vi "Configure Control.vi"(8 "error in (no error)":errorcluster, 10 "control":refnum<vi>, 11 "NT Enum in":refnum<class "NT Enum.lvclass">) -> (0 "error out":errorcluster, 2 "control out":refnum<vi>, 3 "NT Enum out":refnum<class "NT Enum.lvclass">)   [LabVIEW 2020, in "PV Access.lvlib" / "PV Data.lvlib" / "NT Enum.lvclass"]
doc: "Set the description of <B>control</B> from the value's metadata."
uses:
  NT Enum.lvclass
  NT Base/NT Base.lvclass
  NT Enum.lvclass/NT Enum.ctl
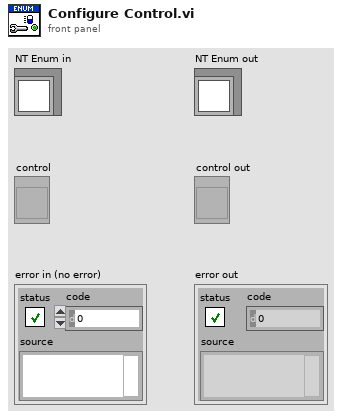
[diagram p1: front panel]
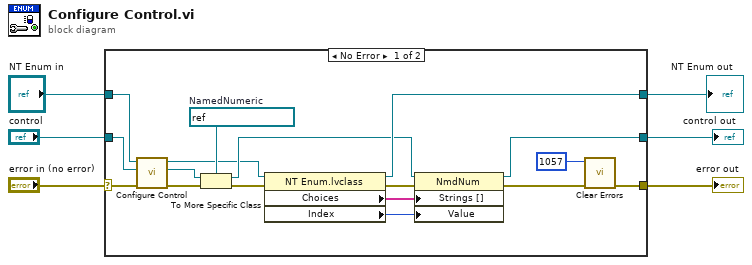
[diagram p0: block diagram]
diagram:
  n1 = case shown="No Error" "error in (no error)" {
    selector: "error in (no error)" -> [w18 w26]
    tunnel: [w9 w26] -> w5
    tunnel: "control" -> [w16 w25]
    tunnel: [w20 w25] -> w3
    tunnel: "NT Enum in" -> [w17 w24]
    tunnel: [w19 w24] -> w1
    frame No Error {
      w12 = refnum<vi> refnum  # NamedNumeric
      n2 = call-parent "Configure Control.vi"("error in (no error)"=w18, "control"=w16, "Base in"=w17) -> ("error out"=w15:errorcluster, "control out"=w13:refnum<vi>, "Base out"=w7:refnum<class "NT Enum.lvclass">)  [unwired: 6 in]
      n3 = To More Specific Class(target class=w12, reference=w13, error in=w15) -> (specific class reference=w11:refnum<vi>, error out=w14:errorcluster)
      n4 = property class="NT Enum.lvclass"(reference=w7, error in=w14) -> (reference out=w19:refnum<class "NT Enum.lvclass">, error out=w23:errorcluster, "Choices"=w22:string[], "Index"=w21:i32)
      n5 = property class="NmdNum"(reference=w11, error in=w23, "Strings []"=w22, "Value"=w21) -> (reference out=w20:refnum<vi>, error out=w10:errorcluster)
      n6 = call <vilib>:"Clear Errors.vi"("error in (no error)"=w10, "specific error code to clear (0: all)"=1057) -> ("error out"=w9:errorcluster)  [unwired: 4 in, 1 out]
    }
    frame Error {
    }
  }
  "error out" <- w5
  "NT Enum out" <- w1
  "control out" <- w3
